vi "TDMS_Open_process.vi"(9 "Input 2D":dbl[][](array[numeric]), 11 "Open":bool) -> (1 "Output 2D":dbl[][](array[numeric]), 3 "Freq_Sampling_SizeX_SizeY":dbl[](array[numeric]))   [LabVIEW 2012]
uses:
  <vilib>/Platform/NI_3dgraph.lvlib
panel:
  in  "3D Surface":refnum<k7>(container)
  in  "Gate 1":dbl
  in  "Gate 2":dbl=25.0
  in  "Samples per Channel":i32=1000 caption="Samples"
  in  "Rate":dbl=60000.0 caption="Sample Rate (Hz)" format="%0.0f"
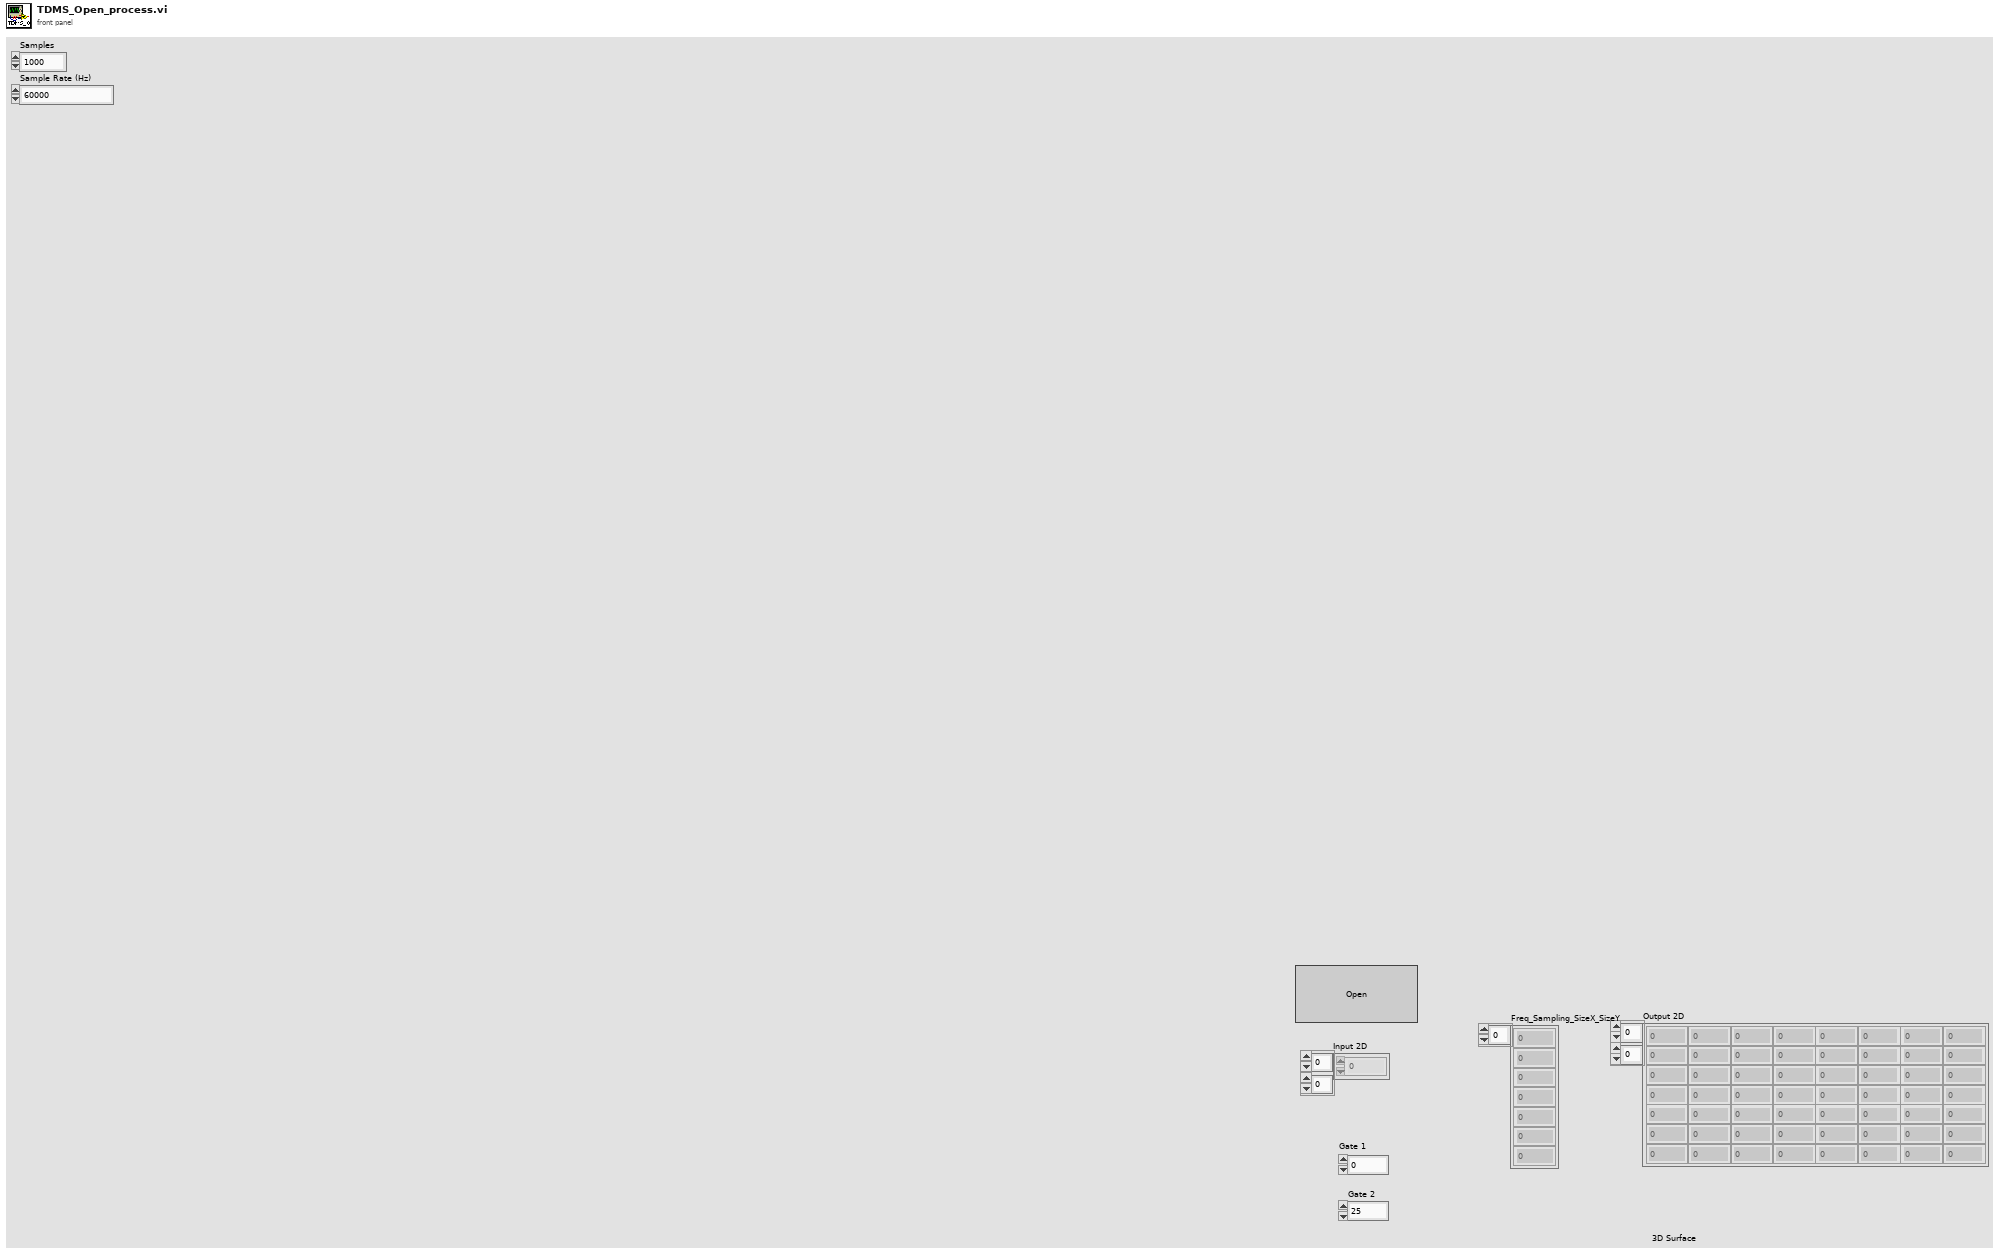
[diagram p1: front panel]
types:
  T1 = enum16{"open", "open or create", "create or replace", "create", "open (read-only)"}
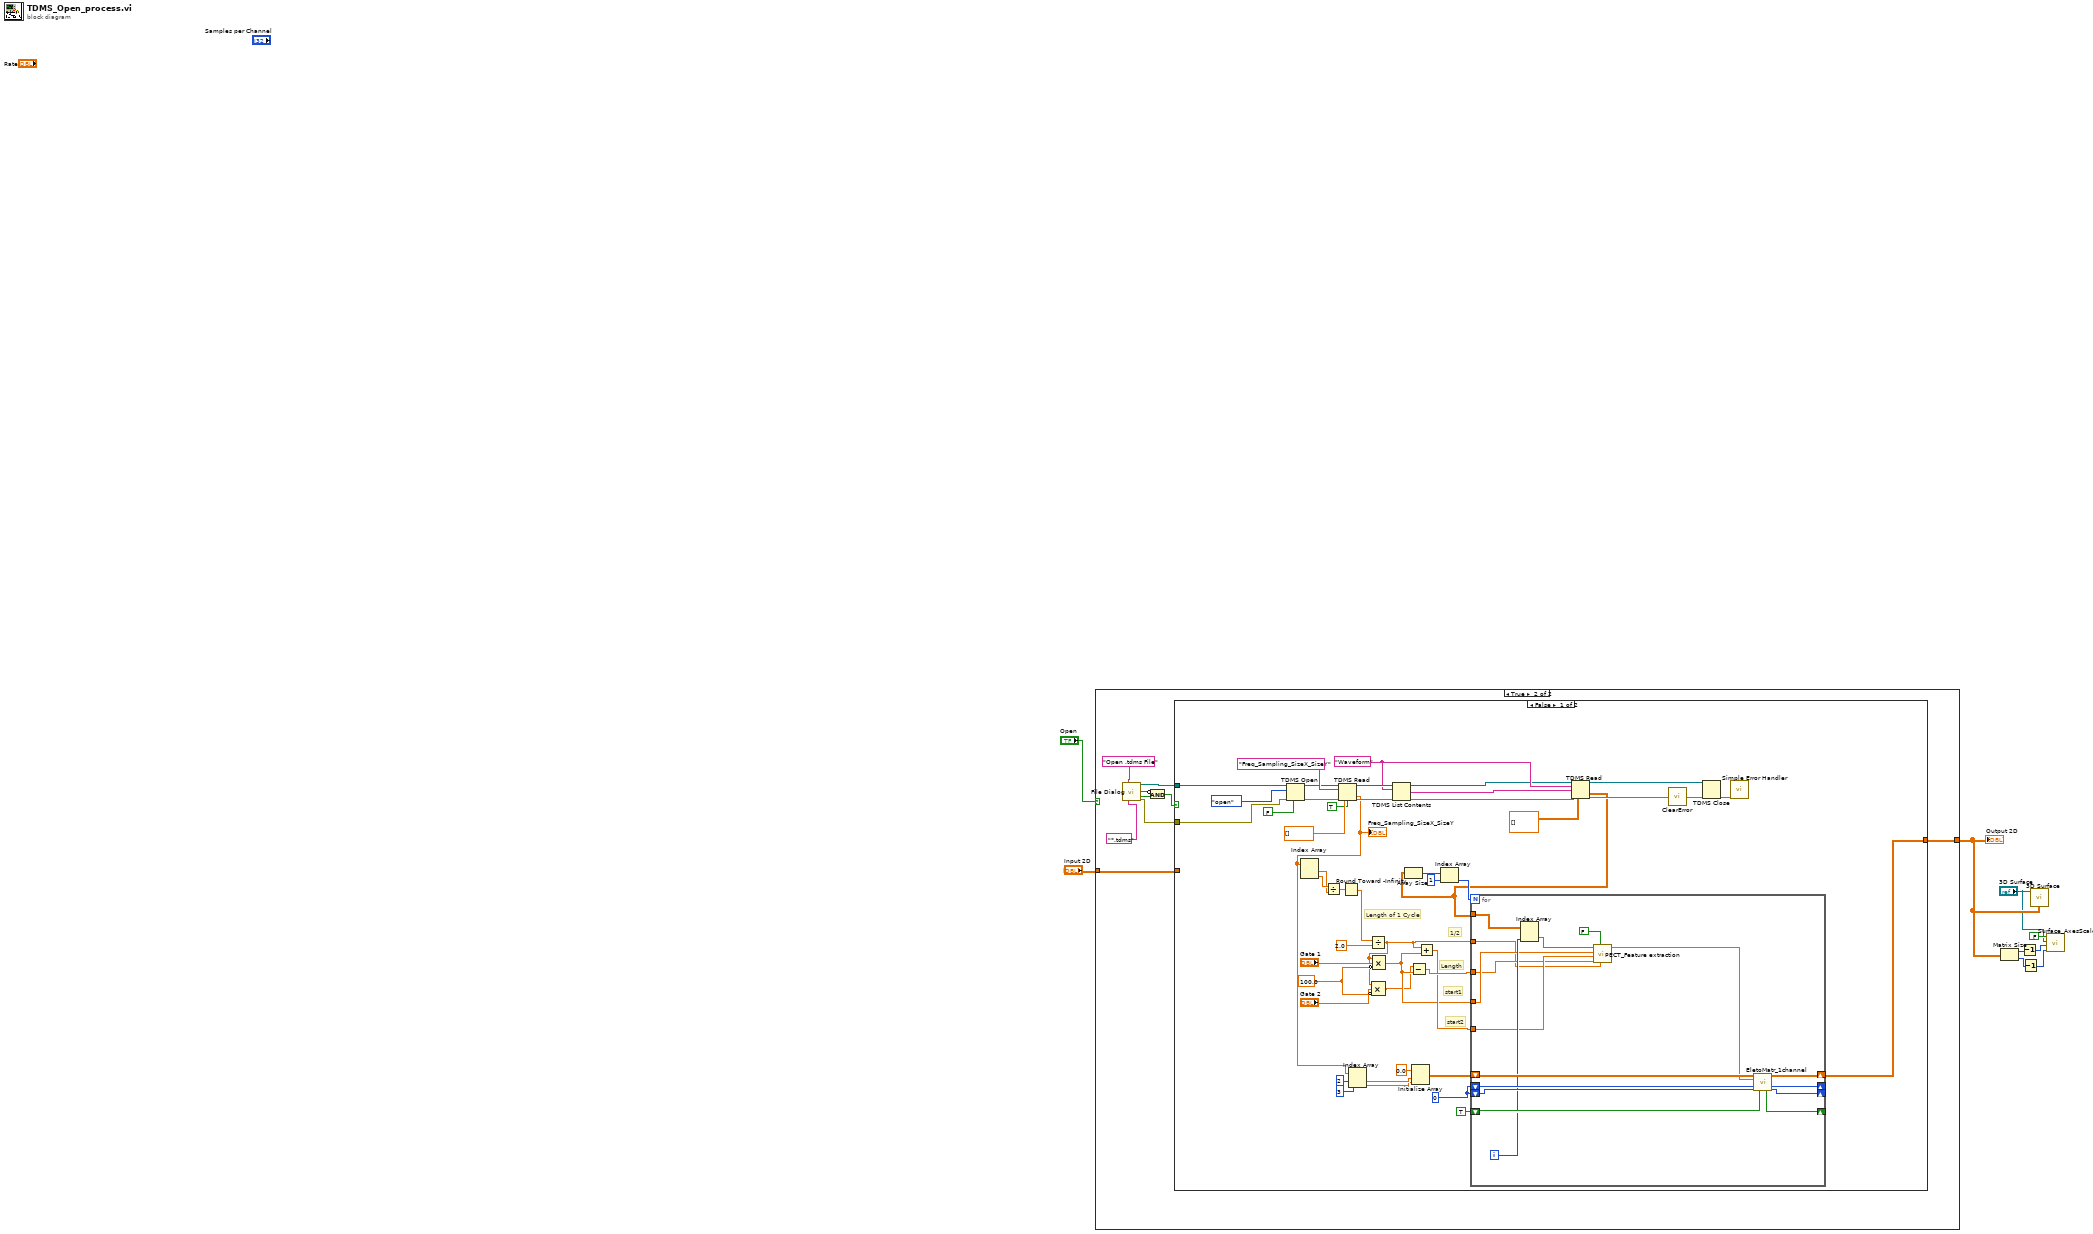
[diagram p0: block diagram]
diagram:
  n1 = case shown="True" "Open" {
    tunnel: [w10 w13] -> w2
    tunnel: "Input 2D" -> [w10 w12]
    frame False {
    }
    frame True {
      n2 = call "File Dialog"("prompt"="Open .tdms File" ("button label"), "pattern (all files)"="*.tdms") -> ("selected path"=w19:path, "exists"=w17:bool, "cancelled"=w16:bool, "error out"=w11:errorcluster)  [unwired: 10 in]
      n3 = Compound Arithmetic op=AND(invert w17, w16) -> (w15:bool)
      n4 = case shown="False" w15 {
        tunnel: w19 -> [w57 _]
        tunnel: [w20 w84] -> w13
        tunnel: w12 -> [_ w84]
        tunnel: w11 -> [w32 _]
        frame False {
          w37 = 100.0 ("蔼")
          w53 = 0 ("Out Row")
          w45 = "Waveform" ("group name in")
          # "Length of 1 Cycle"
          # "start2"
          # "1/2"
          # "start1"
          # "Length"
          n5 = TDMS Open(6:FALSE ("disable buffering (T)"), 8:w32, 10:T1."open" ("operation"), 11:w57) -> (0:w61:errorcluster, 3:w65:refnum<k34>)  [unwired: 2 in]
          n6 = TDMS Read(0:w65, 5:"Freq_Sampling_SizeX_SizeY" ("group name in"), 11:w61, 12:dbl[] [] ("Array"), 13:TRUE ("return channels in file order? (F)")) -> (4:w46:refnum<k34>, 10:w23:dbl[], 15:w31:errorcluster)  [unwired: 3 in, 3 out]
          "Freq_Sampling_SizeX_SizeY" <- w23
          n7 = Index Array(array=w23) -> (element #1=w49:dbl, element #2=w50:dbl)  [unwired: 2 in]
          n8 = Divide(x=w50, y=w49) -> (x/y=w51:dbl)
          n9 = Round Toward -Infinity(1:w51) -> (0:w39:dbl)
          n10 = Index Array(array=w23, index #1=2 ("index"), index #2=3 ("index")) -> (element #1=w22:dbl, element #2=w21:dbl)
          n11 = Divide(x=w39, y=2.0) -> (x/y=w35:dbl)
          n12 = Compound Arithmetic op=MULTIPLY(w35, "Gate 2", invert w37) -> (w36:dbl)
          n13 = Compound Arithmetic op=MULTIPLY(w35, "Gate 1", invert w37) -> (w40:dbl)
          n14 = TDMS List Contents(4:w31, 6:w45, 7:w46) -> (0:w30:errorcluster, 1:w34:string[], 3:w33:refnum<k34>)  [unwired: 1 out]
          n15 = Subtract(x=w36, y=w40) -> (x-y=w55:dbl)
          n16 = Initialize Array(0.0 ("element"), w22, w21) -> (w27:dbl[][])
          n17 = Add(x=w35, y=w40) -> (x+y=w54:dbl)
          n18 = TDMS Read(0:w33, 5:w45, 7:w34, 11:w30, 12:dbl[][] [] ("Array")) -> (4:w48:refnum<k34>, 10:w28:dbl[][], 15:w47:errorcluster)  [unwired: 3 in, 3 out]
          n19 = Array Size(array=w28) -> (size(s)=w44:i32[])
          n20 = Index Array(array=w44, index=1) -> (element=w42:i32)
          n21 = for {
            N: w42 -> [_]
            tunnel: w55 -> [w71]
            tunnel: w54 -> [w72]
            tunnel: w40 -> [w73]
            tunnel: w35 -> [w70]
            shift-right: [w82] -> w20
            shift-left: w27 -> [w83]
            shift-right: [w81] -> _
            shift-left: w53 -> [w78]
            shift-right: [w80] -> _
            shift-left: w53 -> [w79]
            shift-right: [w76] -> _
            shift-left: TRUE ("Output Direction") -> [w77]
            tunnel: w28 -> [w75]
            i -> [w74]
            n22 = Index Array(array=w75, index (col)=w74) -> (element=w67:dbl[])  [unwired: 1 in]
            n23 = call "PECT_Feature extraction.vi"("Length T/2"=w70, "Offset"=FALSE, "Length"=w71, "Start 2"=w72, "Start 1"=w73, "Pulse signal in"=w67) -> ("Feature extraction out"=w68:dbl)  [unwired: 5 in]
            n24 = call "EletoMatr_1channel.vi"("Input Array X"=w83, "Input data"=w68, "In Row"=w78, "In Column"=w79, "Input Direction"=w77) -> ("Out Array X"=w82:dbl[][], "Out Row"=w81:i32, "Output Direction"=w76:bool, "Out Column"=w80:i32)  [unwired: 6 in, 1 out]
          }
          n25 = call <vilib>:"ClearError.vi"("error in (no error)"=w47) -> ("error out"=w59:errorcluster)
          n26 = TDMS Close(8:w59, 11:w48) -> (0:w58:errorcluster)  [unwired: 1 out]
          n27 = call <vilib>:"Simple Error Handler.vi"("error in (no error)"=w58) -> ()  [unwired: 1 in, 8 out]
        }
        frame True {
        }
      }
    }
  }
  "Output 2D" <- w2
  n28 = Matrix Size(0:w2) -> (1:w3:i32, 2:w4:i32)
  n29 = Decrement(x=w3) -> (x-1=w7:i32)
  n30 = Decrement(x=w4) -> (x-1=w6:i32)
  n31 = call <vilib>:"3D Surface.vi"("z matrix"=w2, "3D graph"="3D Surface") -> ()  [unwired: 8 in, 2 out]
  n32 = call "Surface_AxesScale.vi"("Y-axis Max"=w6, "X-axis max"=w7, "3D Surface"="3D Surface", "Auto Scale"=FALSE) -> ()  [unwired: 8 in]
